vi "Delete Value.vi"(8 "error in (no error)":errorcluster, 10 "Key":i32, 11 "Integer Dictionary in":refnum<class "Integer Dictionary.lvclass">) -> (0 "error out":errorcluster, 2 "found?":bool, 3 "Integer Dictionary out":refnum<class "Integer Dictionary.lvclass">)   [LabVIEW 2020, in "Integer Dictionary.lvclass"]
uses:
  Integer Dictionary.lvclass
  Integer Dictionary.lvclass/Integer Dictionary.ctl
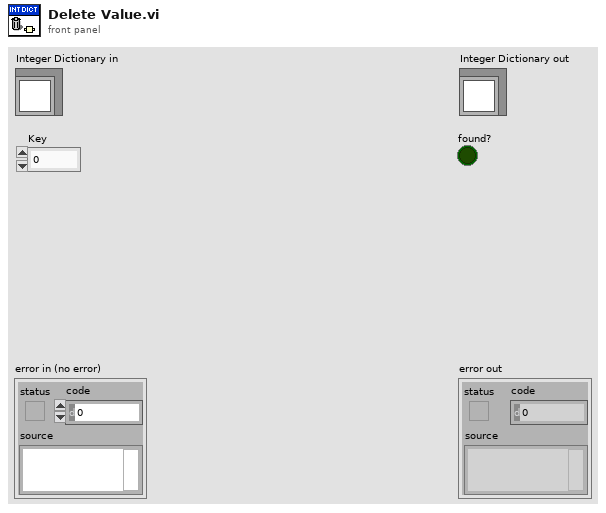
[diagram p1: front panel]
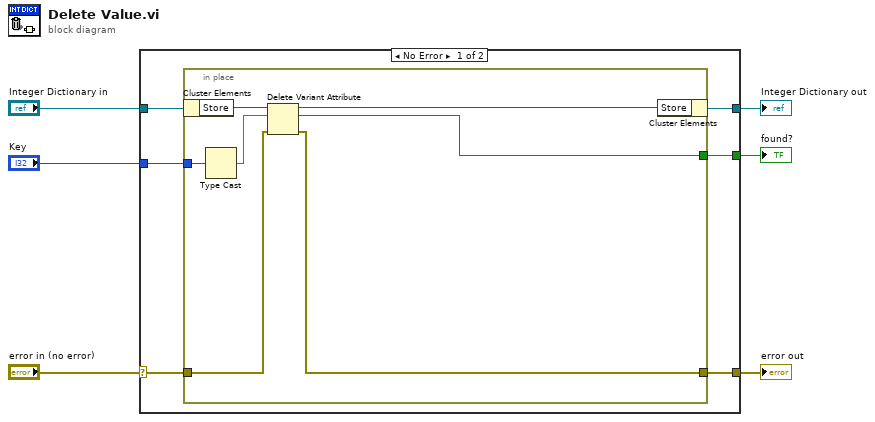
[diagram p0: block diagram]
diagram:
  n1 = case shown="No Error" "error in (no error)" {
    selector: "error in (no error)" -> [w10 w21]
    tunnel: [w9 w21] -> w5
    tunnel: [w11 w20] -> w3
    tunnel: "Integer Dictionary in" -> [w12 w20]
    tunnel: "Key" -> [w8 _]
    tunnel: [w7 _] -> w1
    frame No Error {
      n2 = in-place {
        in-place-border: w10 -> [w18]
        in-place-border: [w17] -> w9
        in-place-border: w8 -> [w16]
        in-place-border: [w13] -> w7
        n3 = in-place-cluster #1(w12) -> ("Store"=w19:variant)
        n4 = Type Cast(x=w16) -> (*(type *) &x=w15:string)  [unwired: 1 in]
        n5 = Delete Variant Attribute(4:w18, 6:w15, 7:w19) -> (0:w17:errorcluster, 2:w13:bool, 3:w14:variant)
        n6 = in-place-cluster #1("Store"=w14) -> (w11:refnum<class "Integer Dictionary.lvclass">)
      }
    }
    frame Error {
    }
  }
  "error out" <- w5
  "Integer Dictionary out" <- w3
  "found?" <- w1
